vi "Write Control Value to Cam.vi"(8 "error in (no error)":errorcluster, 11 "Camera Settings Dialog in":refnum<class "Camera Settings Dialog.lvclass">) -> (0 "error out":errorcluster, 3 "Camera Settings Dialog out":refnum<class "Camera Settings Dialog.lvclass">)   [LabVIEW 2020, in "Camera Settings Dialog UI.lvlib" / "Camera Settings Dialog.lvclass"]
uses:
  Camera Settings Dialog.lvclass
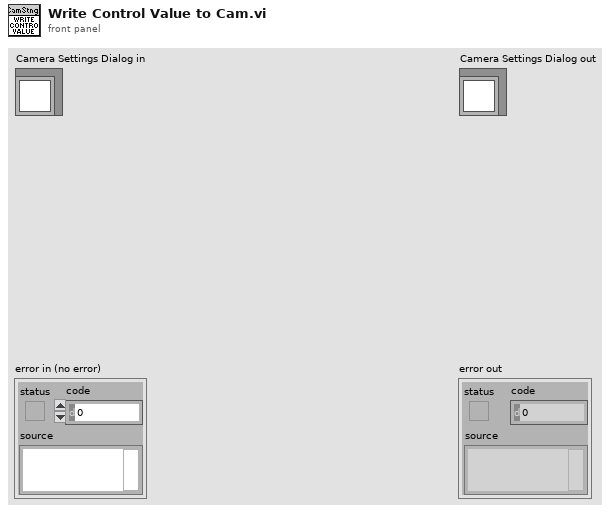
[diagram p1: front panel]
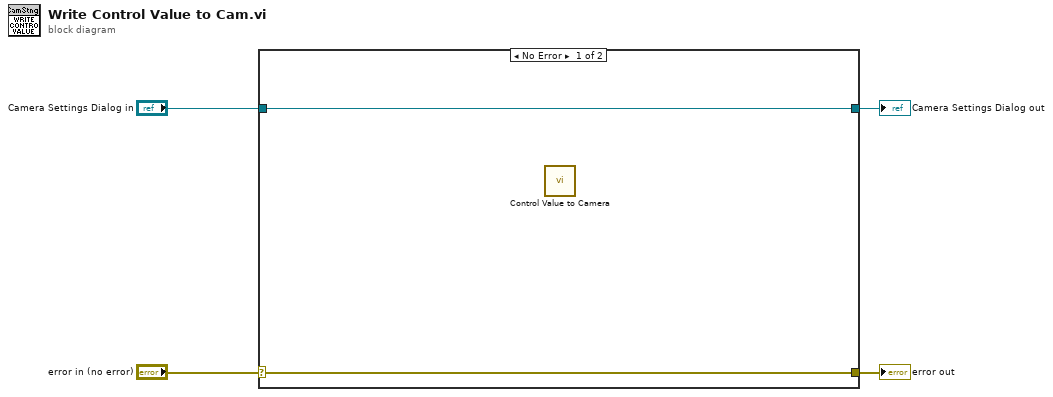
[diagram p0: block diagram]
diagram:
  n1 = case shown="No Error" "error in (no error)" {
    selector: "error in (no error)" -> [w5 w8]
    tunnel: [w5 w8] -> w3
    tunnel: [w6 w7] -> w1
    tunnel: "Camera Settings Dialog in" -> [w6 w7]
    frame No Error {
      n2 = call "Control Value to Camera.vi"() -> ()  [unwired: 6 in, 2 out]
    }
    frame Error {
    }
  }
  "error out" <- w3
  "Camera Settings Dialog out" <- w1
